vi "Periodic Tasks.vi"(8 "error in":errorcluster) -> ()   [LabVIEW 2012]
doc: "This VI runs in parallel to other tasks. It can contain as many user-defined periodic loops as you need. These can carry out PID or other sorts of timed response."
uses:
  <vilib>/Rock Robotics/WPI/DriverStation/DriverStationLCD/WPI_DriverStationLCDLCDLine.ctl
  <vilib>/Rock Robotics/SystemInterfaces/Utilities/FPGA_UtilitiesLED Source.ctl
  <vilib>/Rock Robotics/SystemInterfaces/Utilities/FPGA_UtilitiesLED State.ctl
  Robot Global Data.vi
  <vilib>/Rock Robotics/WPI/Solenoid/Deprecated/WPI_SolenoidSetBool.vi
  <vilib>/Rock Robotics/WPI/Joystick/WPI_JoystickGetSetRefNum.vi
  <vilib>/Rock Robotics/WPI/Compressor/WPI_CompressorGetSetRefNum.vi
  <vilib>/Rock Robotics/WPI/RobotDrive/WPI_RobotDriveGetSetRefNum.vi
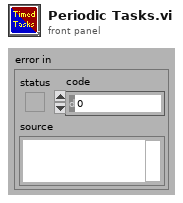
[diagram p1: front panel]
types:
  T1 = typedef "FPGA_UtilitiesLED State.ctl" = enum16{"Off", "On", "Toggle"}
  T2 = typedef "FPGA_UtilitiesLED Source.ctl" = enum16{"User LED", "FPGA LED"}
  T3 = typedef "WPI_CompressorDevRef.ctl" = cluster{"DevStatus":errorcluster, "DigitalInputDevRef":T4, "RelayDevRef":T7}
  T4 = typedef "WPI_DigitalInputDevRef.ctl" = cluster{"DevStatus":errorcluster, "DIO Channel":T5, "Digital Module":T6}
  T5 = typedef "FPGA_DIOChannel.ctl" = enum8{"DIO 1", "DIO 2", "DIO 3", "DIO 4", "DIO 5", "DIO 6", "DIO 7", "DIO 8", "DIO 9", "DIO 10", "DIO 11", "DIO 12", "DIO 13", "DIO 14", "Invalid"}
  T6 = typedef "FPGA_TypedefDigitalModule.ctl" = enum16{"Digital Module 1", "Digital Module 2"}
  T7 = typedef "WPI_RelayDevRef.ctl" = cluster{"DevStatus":errorcluster, "Relay Channel":T8, "Digital Module":T6, "Relay Direction":T9}
  T8 = typedef "FPGA_DIORelayChannel.ctl" = enum8{"Relay 1", "Relay 2", "Relay 3", "Relay 4", "Relay 5", "Relay 6", "Relay 7", "Relay 8", "Invalid"}
  T9 = typedef "WPI_RelayDirection.ctl" = enum16{"Both directions", "Forward only", "Reverse only"}
  T10 = typedef "WPI_EncoderDevRef.ctl" = cluster{"DevStatus":errorcluster, "EncoderIndex":T11, "CounterIndex":T12, "DistancePerCount":dbl, "Decoding Type":T13}
  T11 = typedef "FPGA_EncoderIdx.ctl" = enum8{"Enc 0", "Enc 1", "Enc 2", "Enc 3", "Invalid"}
  T12 = typedef "FPGA_CounterCtrSystemIndex.ctl" = enum8{"Ctr 0", "Ctr 1", "Ctr 2", "Ctr 3", "Ctr 4", "Ctr 5", "Ctr 6", "Ctr 7", "Invalid"}
  T13 = typedef "WPI_EncoderType.ctl" = enum16{"1x", "2x", "4x"}
  T14 = typedef "WPI_JoystickDevRef.ctl" = cluster{"Device":T15}
  T15 = typedef "WPI_JoystickDeviceEnum.ctl" = enum16{"USB 1", "USB 2", "USB 3", "USB 4", "Kinect 1", "Kinect 2"}
  T16 = typedef "WPI_RobotDriveDevRef.ctl" = cluster{"DevStatus":errorcluster, "Motors[]":T17[], "Square Inputs":bool, "Max Output":dbl, "Isochronous":bool}
  T17 = typedef "WPI_MotorControlDeviceRef.ctl" = cluster{"DeviceStatus":errorcluster, "Type":enum16{"PWM", "CAN"}, "PWM":cluster{"Digital Module":T6, "PWM Channel":T18, "DeadBand":T19}, "CAN":cluster{"Device Number":u8, "Control Mode":T20, "Semaphore":T21, "Max Vout":dbl}, "Invert":bool, "TransformRef":T22, "InvTransformRef":T22}
  T18 = typedef "FPGA_DIOPWMChannel.ctl" = enum8{"PWM 1", "PWM 2", "PWM 3", "PWM 4", "PWM 5", "PWM 6", "PWM 7", "PWM 8", "PWM 9", "PWM 10", "Invalid"}
  T19 = typedef "WPI_PWMDeadband.ctl" = cluster{"Name":string, "maxPositivePwm":i32, "minPositivePwm":i32, "centerPwm":i32, "maxNegativePwm":i32, "minNegativePwm":i32, "angularRange":u16}
  T20 = typedef "WPI_CANJaguar_ControlMode.ctl" = enum8{"Percent VBus", "Current", "Speed", "Position", "Voltage"}
  T21 = typedef "Semaphore RefNum" = refnum<k1>
  T22 = typedef "WPI_PWMTransform_ConPane.ctl" = refnum<vi>
  T23 = typedef "WPI_DriverStationLCDLCDLine.ctl" = enum16{"Main - Line 1", "User - Line 2", "User - Line 3", "User - Line 4", "User - Line 5", "User - Line 6"}
  T24 = typedef "WPI_SolenoidDevRef.ctl" = cluster{"DevStatus":errorcluster, "Solenoid Module":T25, "Forward Solenoid Channel":T26, "Reverse Solenoid Channel":T26}
  T25 = typedef "FPGA_TypedefSolenoidModule.ctl" = enum16{"Solenoid Module 1", "Solenoid Module 2"}
  T26 = typedef "WPI_SolenoidChannel.ctl" = enum8{"Solenoid 1", "Solenoid 2", "Solenoid 3", "Solenoid 4", "Solenoid 5", "Solenoid 6", "Solenoid 7", "Solenoid 8", "Invalid"}
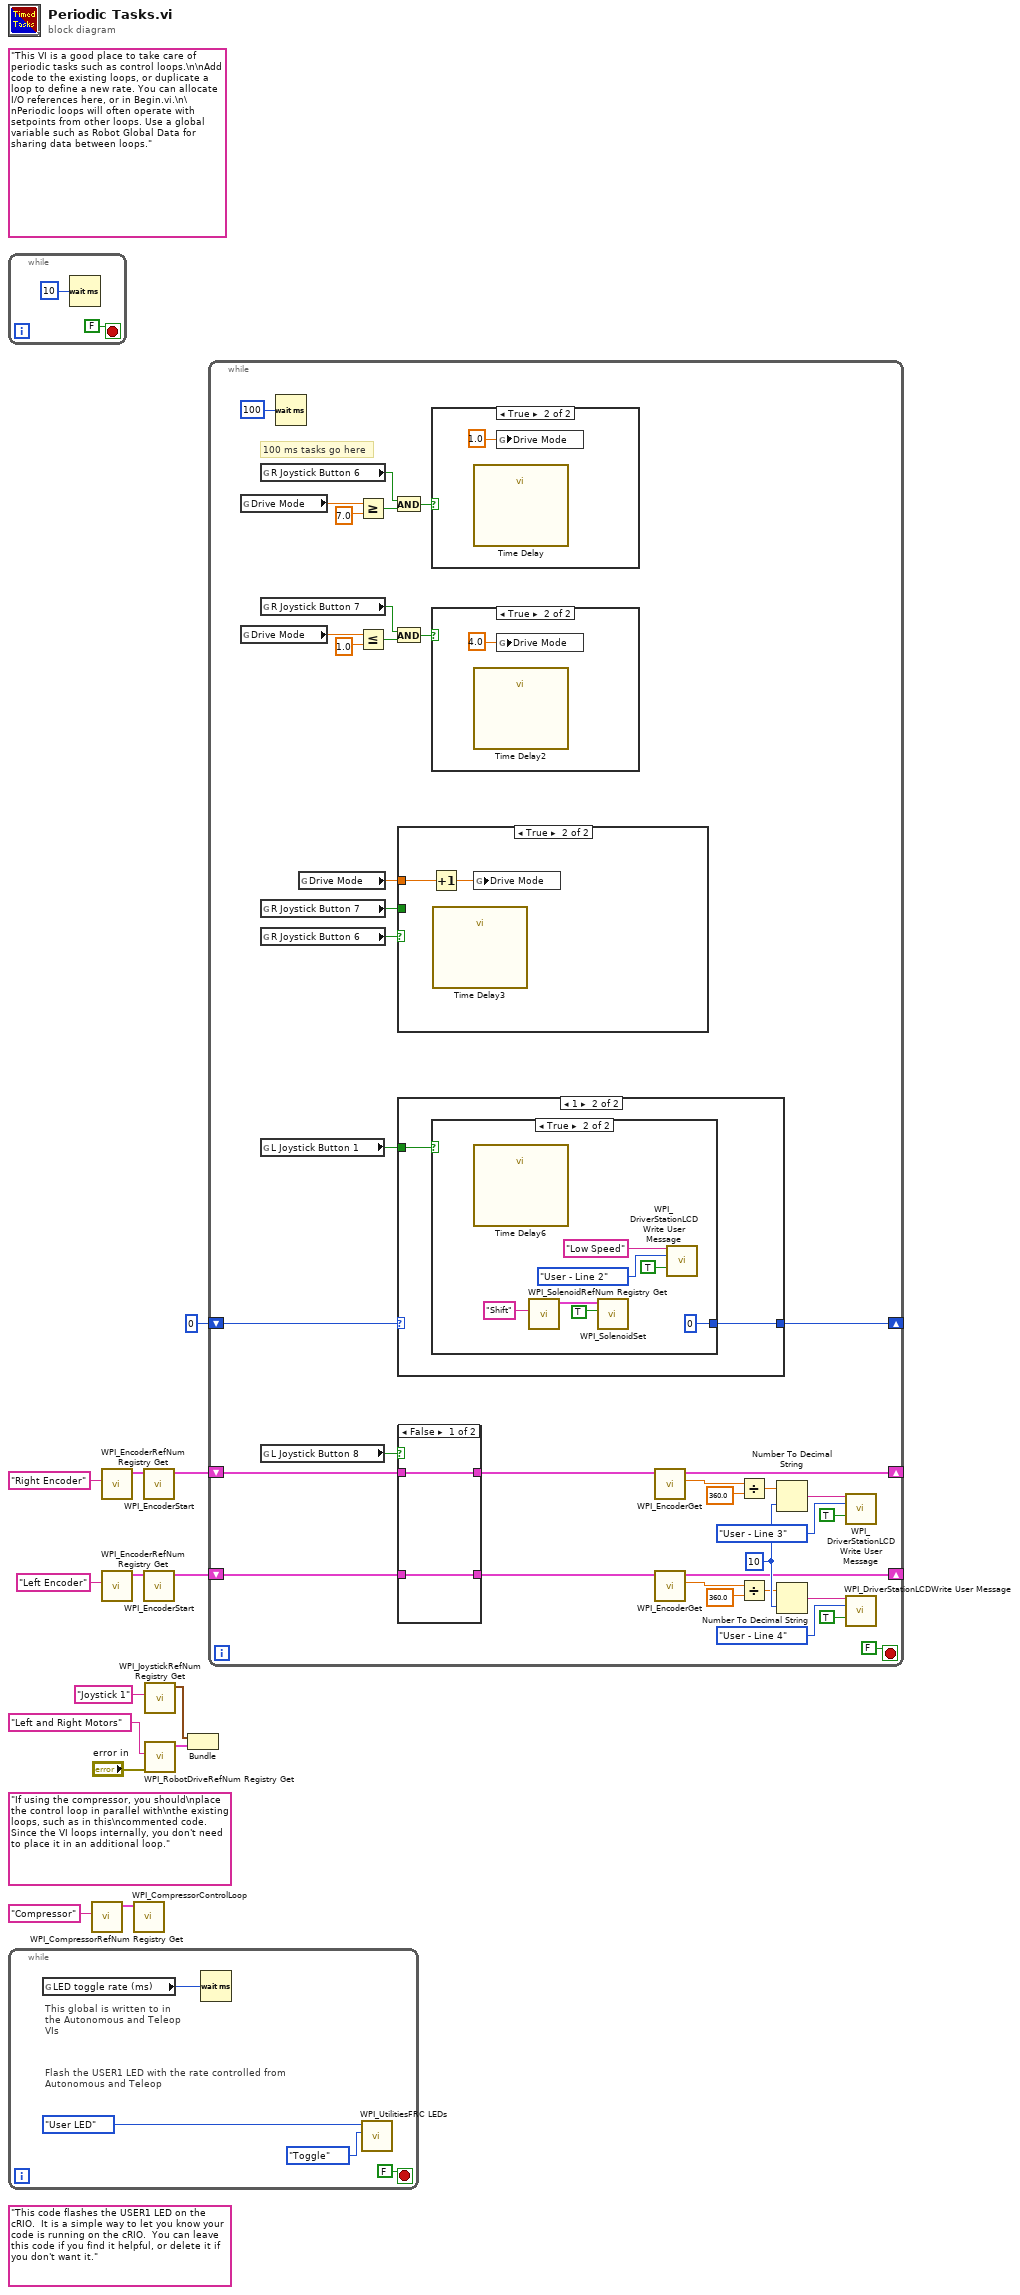
[diagram p0: block diagram]
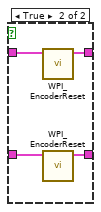
[diagram p2: hidden frame]
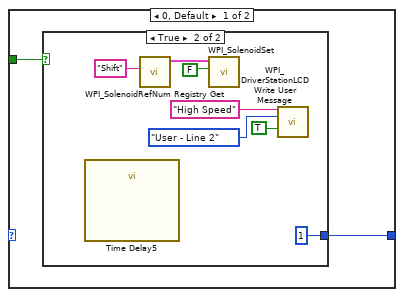
[diagram p3: hidden frame]
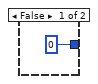
[diagram p4: hidden frame]
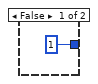
[diagram p5: hidden frame]
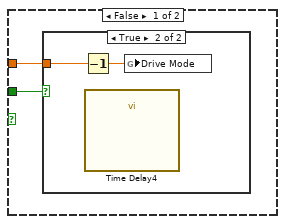
[diagram p6: hidden frame]
diagram:
  (unwired) "If using the compressor, you should\nplace the control loop in parallel with\nthe existing loops, such as in this\ncommented code. Since the VI loops internally, you don't need to place it in an additional loop."
  (unwired) "This code flashes the USER1 LED on the cRIO.  It is a simple way to let you know your code is running on the cRIO.  You can leave this code if you find it helpful, or delete it if you don't want it."
  (unwired) "This VI is a good place to take care of periodic tasks such as control loops.\n\nAdd code to the existing loops, or duplicate a loop to define a new rate. You can allocate I/O references here, or in Begin.vi.\n\nPeriodic loops will often operate with setpoints from other loops. Use a global variable such as Robot Global Data for sharing data between loops."
  n1 = while {
    stop <- FALSE stop-if-true
    n2 = Wait (ms)(milliseconds to wait=u32 10) -> ()  [unwired: 1 out]
  }
  n3 = while {
    stop <- FALSE stop-if-true
    # "This global is written to in the Autonomous and Teleop VIs"
    # "Flash the USER1 LED with the rate controlled from Autonomous and Teleop"
    n4 = global read "Robot Global Data.vi" "LED toggle rate (ms)"() -> (w17:u32)
    n5 = Wait (ms)(milliseconds to wait=w17) -> ()  [unwired: 1 out]
    n6 = call <vilib>:"WPI_UtilitiesFRC LEDs.vi"("State"=FPGA_UtilitiesLED_State."Toggle", "LED Type"=FPGA_UtilitiesLED_Source."User LED") -> ()  [unwired: 1 in, 9 out]
  }
  n7 = call <vilib>:"WPI_CompressorRefNum Registry Get.vi"("refnum name"="Compressor") -> ("CompressorDevRef"=w13:T3)  [unwired: 9 in, 1 out]
  n8 = call <vilib>:"WPI_EncoderRefNum Registry Get.vi"("refnum name"="Right Encoder") -> ("EncoderDevRef"=w5:T10)  [unwired: 9 in, 1 out]
  n9 = call <vilib>:"WPI_EncoderRefNum Registry Get.vi"("refnum name"="Left Encoder") -> ("EncoderDevRef"=w6:T10)  [unwired: 9 in, 1 out]
  n10 = call <vilib>:"WPI_CompressorControlLoop.vi"("CompressorDevRef"=w13) -> ()  [unwired: 11 in]
  n11 = call <vilib>:"WPI_EncoderStart.vi"("EncoderDevRef"=w5) -> ("EncoderDevRef"=w2:T10)  [unwired: 9 in, 1 out]
  n12 = call <vilib>:"WPI_EncoderStart.vi"("EncoderDevRef"=w6) -> ("EncoderDevRef"=w1:T10)  [unwired: 9 in, 1 out]
  n13 = call <vilib>:"WPI_JoystickRefNum Registry Get.vi"("refnum name"="Joystick 1") -> ("JoystickDevRef"=w10:T14)  [unwired: 1 in, 9 out]
  n14 = call <vilib>:"WPI_RobotDriveRefNum Registry Get.vi"("error in (no error)"="error in", "refnum name"="Left and Right Motors") -> ("RobotDriveDevRef"=w9:T16)  [unwired: 9 out]
  n15 = Bundle("JoystickDevRef"=w10, "RobotDriveDevRef"=w9) -> ()  [unwired: 2 out]
  n16 = while {
    shift-right: [w42] -> _
    shift-left: 0 -> [w41]
    shift-right: [w28] -> _
    shift-left: w2 -> [w30]
    shift-right: [w27] -> _
    shift-left: w1 -> [w29]
    stop <- FALSE stop-if-true
    w40 = i16 10 ("width (-)")
    # "100 ms tasks go here"
    n17 = global read "Robot Global Data.vi" "Drive Mode"() -> (w56:dbl)
    n18 = global read "Robot Global Data.vi" "Drive Mode"() -> (w51:dbl)
    n19 = global read "Robot Global Data.vi" "R Joystick Button 6"() -> (w54:bool)
    n20 = global read "Robot Global Data.vi" "R Joystick Button 7"() -> (w49:bool)
    n21 = global read "Robot Global Data.vi" "R Joystick Button 7"() -> (w44:bool)
    n22 = global read "Robot Global Data.vi" "R Joystick Button 6"() -> (w46:bool)
    n23 = global read "Robot Global Data.vi" "L Joystick Button 1"() -> (w43:bool)
    n24 = global read "Robot Global Data.vi" "L Joystick Button 8"() -> (w31:bool)
    n25 = Wait (ms)(milliseconds to wait=u32 100) -> ()  [unwired: 1 out]
    n26 = global read "Robot Global Data.vi" "Drive Mode"() -> (w45:dbl)
    n27 = Greater Or Equal?(x=w56, y=7.0) -> (x >= y?=w53:bool)
    n28 = Less Or Equal?(x=w51, y=1.0) -> (x <= y?=w48:bool)
    n29 = And(x=w54, y=w53) -> (x .and. y?=w52:bool)
    n30 = And(x=w49, y=w48) -> (x .and. y?=w47:bool)
    n31 = case shown="True" w46 {
      tunnel: w45 -> [w85 w90]
      tunnel: w44 -> [w86 _]
      frame False {
        n32 = case shown="True" w86 {
          tunnel: w85 -> [_ w87]
          frame False {
          }
          frame True {
            n33 = Decrement(x=w87) -> (x-1=w88:dbl)
            n34 = call "Time Delay4"() -> ()  [unwired: 11 in, 1 out]
            n35 = global write "Robot Global Data.vi" "Drive Mode"(w88) -> ()
          }
        }
      }
      frame True {
        n36 = Increment(x=w90) -> (x+1=w89:dbl)
        n37 = call "Time Delay3"() -> ()  [unwired: 11 in, 1 out]
        n38 = global write "Robot Global Data.vi" "Drive Mode"(w89) -> ()
      }
    }
    n39 = case shown="1" w41 {
      tunnel: [w65 w75] -> w42
      tunnel: w43 -> [w66 w76]
      frame 0, Default {
        n40 = case shown="True" w66 {
          tunnel: [0 1] -> w65
          frame False {
          }
          frame True {
            n41 = call "Time Delay5"() -> ()  [unwired: 11 in, 1 out]
            n42 = call <vilib>:"WPI_SolenoidRefNum Registry Get.vi"("refnum name"="Shift") -> ("SolenoidDevRef"=w72:T24)  [unwired: 9 in, 1 out]
            n43 = call-poly <vilib>:"WPI_SolenoidSet.vi"("Value"=FALSE, "SolenoidDevRef"=w72) -> ()  [unwired: 8 in, 2 out]
            n44 = call <vilib>:"WPI_DriverStationLCDWrite User Message.vi"("line text"="High Speed", "line"=WPI_DriverStationLCDLCDLine."User - Line 2", "clear line before write (T)"=TRUE) -> ()  [unwired: 12 in, 1 out]
          }
        }
      }
      frame 1 {
        n45 = case shown="True" w76 {
          tunnel: [1 0] -> w75
          frame False {
          }
          frame True {
            n46 = call "Time Delay6"() -> ()  [unwired: 11 in, 1 out]
            n47 = call <vilib>:"WPI_SolenoidRefNum Registry Get.vi"("refnum name"="Shift") -> ("SolenoidDevRef"=w82:T24)  [unwired: 9 in, 1 out]
            n48 = call-poly <vilib>:"WPI_SolenoidSet.vi"("Value"=TRUE, "SolenoidDevRef"=w82) -> ()  [unwired: 8 in, 2 out]
            n49 = call <vilib>:"WPI_DriverStationLCDWrite User Message.vi"("line text"="Low Speed", "line"=WPI_DriverStationLCDLCDLine."User - Line 2", "clear line before write (T)"=TRUE) -> ()  [unwired: 12 in, 1 out]
          }
        }
      }
    }
    n50 = case shown="False" w31 {
      tunnel: [w59 w64] -> w32
      tunnel: [w60 w63] -> w33
      tunnel: w30 -> [w60 w62]
      tunnel: w29 -> [w59 w61]
      frame False {
      }
      frame True {
        n51 = call <vilib>:"WPI_EncoderReset.vi"("EncoderDevRef"=w62) -> ("EncoderDevRef"=w63:T10)  [unwired: 9 in, 1 out]
        n52 = call <vilib>:"WPI_EncoderReset.vi"("EncoderDevRef"=w61) -> ("EncoderDevRef"=w64:T10)  [unwired: 9 in, 1 out]
      }
    }
    n53 = case shown="True" w52 {
      frame False {
      }
      frame True {
        n54 = call "Time Delay"() -> ()  [unwired: 11 in, 1 out]
        n55 = global write "Robot Global Data.vi" "Drive Mode"(1.0 ("Drive Mode")) -> ()
      }
    }
    n56 = case shown="True" w47 {
      frame False {
      }
      frame True {
        n57 = call "Time Delay2"() -> ()  [unwired: 11 in, 1 out]
        n58 = global write "Robot Global Data.vi" "Drive Mode"(4.0 ("Drive Mode")) -> ()
      }
    }
    n59 = call <vilib>:"WPI_EncoderGet.vi"("EncoderDevRef"=w33) -> ("Distance"=w24:dbl, "EncoderDevRef"=w28:T10)  [unwired: 5 in, 4 out]
    n60 = call <vilib>:"WPI_EncoderGet.vi"("EncoderDevRef"=w32) -> ("Distance"=w22:dbl, "EncoderDevRef"=w27:T10)  [unwired: 5 in, 4 out]
    n61 = Divide(x=w24, y=360.0) -> (x/y=w23:dbl)
    n62 = Divide(x=w22, y=360.0) -> (x/y=w21:dbl)
    n63 = Number To Decimal String(number=w23, width (-)=w40) -> (decimal integer string=w38:string)
    n64 = Number To Decimal String(number=w21, width (-)=w40) -> (decimal integer string=w39:string)
    n65 = call <vilib>:"WPI_DriverStationLCDWrite User Message.vi"("line text"=w38, "line"=WPI_DriverStationLCDLCDLine."User - Line 3", "clear line before write (T)"=TRUE) -> ()  [unwired: 12 in, 1 out]
    n66 = call <vilib>:"WPI_DriverStationLCDWrite User Message.vi"("line text"=w39, "line"=WPI_DriverStationLCDLCDLine."User - Line 4", "clear line before write (T)"=TRUE) -> ()  [unwired: 12 in, 1 out]
  }
